vi "FaceSymbol2Color.vi"(9 "Pict Ring":T1, 10 "Pict Ring 2":T1, 11 "Array":string[](array[string])) -> (3 "String":string)   [LabVIEW 2017]
uses:
  FaceletColorRing.ctl
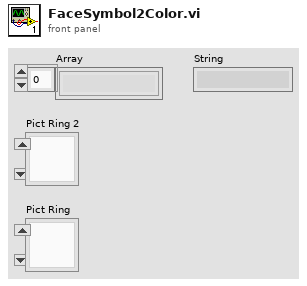
[diagram p1: front panel]
types:
  T1 = typedef "FaceletColorRing.ctl" = u16
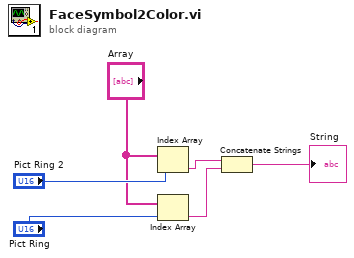
[diagram p0: block diagram]
diagram:
  n1 = Index Array(array="Array", index="Pict Ring 2") -> (element=w4:string)
  n2 = Index Array(array="Array", index="Pict Ring") -> (element=w1:string)
  n3 = Concatenate Strings(w4, w1) -> (→"String":string)
